vi "lab3_usrp_image_transceiver.vi"() -> ()   [LabVIEW 2014]
uses:
  glb_ackTable.vi
  var_stop.vi
  <vilib>/addons/Modulation/niDMT.lvlib
  <vilib>/addons/Modulation/Digital/General/MT Apply Pulse Shaping Filter (Generic).vi
  <vilib>/addons/Modulation/Analog/controls/Complex Data Waveform.ctl
  <vilib>/addons/Modulation/niAMT.lvlib
  <instrlib>/niUSRP/niUSRP Write Tx Data (CDB Cluster).vi
  <instrlib>/niUSRP/niUSRP Fetch Rx Data (CDB Cluster).vi
  <vilib>/addons/Modulation/Digital/General/MT Apply Matched Filter (Generic).vi
  <vilib>/addons/Modulation/Digital/General/MT Align to Ideal Symbols (Generic).vi
  glb_complete.vi
panel:
  in  "Debug":bool
  out "Constellation Graph":cdb[](graph)
  out "RX coerced gain":dbl format="%#_6f"
  out "TX coerced gain":dbl format="%#_6f"
  out "coerced carrier frequency":dbl=100000.0 format="%#_6p"
  out "coerced IQ rate":dbl=100000.0 format="%#_6p"
  out "Download progress":dbl(slide) scale=0.0..100.0
  out "Received Image":picture
  out "total bytes RX":i32
  in  "soft decision?":bool
  in  "RX number of samples":i64=40000
  in  "RX Frequency Source":string(combo)="Internal"
  in  "TX Frequency Source":string(combo)="Internal"
  in  "RX ant gain":dbl format="%#_6f"
  in  "TX ant gain":dbl format="%#_6f"
  in  "carrier frequency":dbl=915000000.0 format="%#_6p"
  in  "IQ rate":dbl=800000.0 format="%#_6p"
  in  "RX antenna name":string="RX2"
  in  "TX antenna name":string="TX1"
  in  "RX device names":refnum<k15>="192.168.10.2"
  in  "TX device names":refnum<k15>="192.168.10.2"
  in  "filter length (symbols)":i32=11
  in  "filter parameter":dbl=0.35 format="%.2f"
  in  "pulse shaping filter (none)":T1(ring)=enum."Root Raised Cos"
  in  "samples per symbol (16)":i32=4
  in  "Tab Control":T2(tab)=enum."r=1/2 (13,17)"
  in  "modulation 2":enum16{"BPSK", "QPSK"}(ring)
  in  "modulation 3":enum16{"BPSK", "QPSK"}(ring)=enum."QPSK"
  in  "modulation":enum16{"BPSK", "QPSK", "16QAM"}(ring)
  in  "stop":bool
  out "Length of last packet":i32
  out "total packets":dbl
  in  "bytes per packet":i32=1000
  out "Original image":picture
  out "Total bits TX":i32
  in  "file path (use dialog)":path
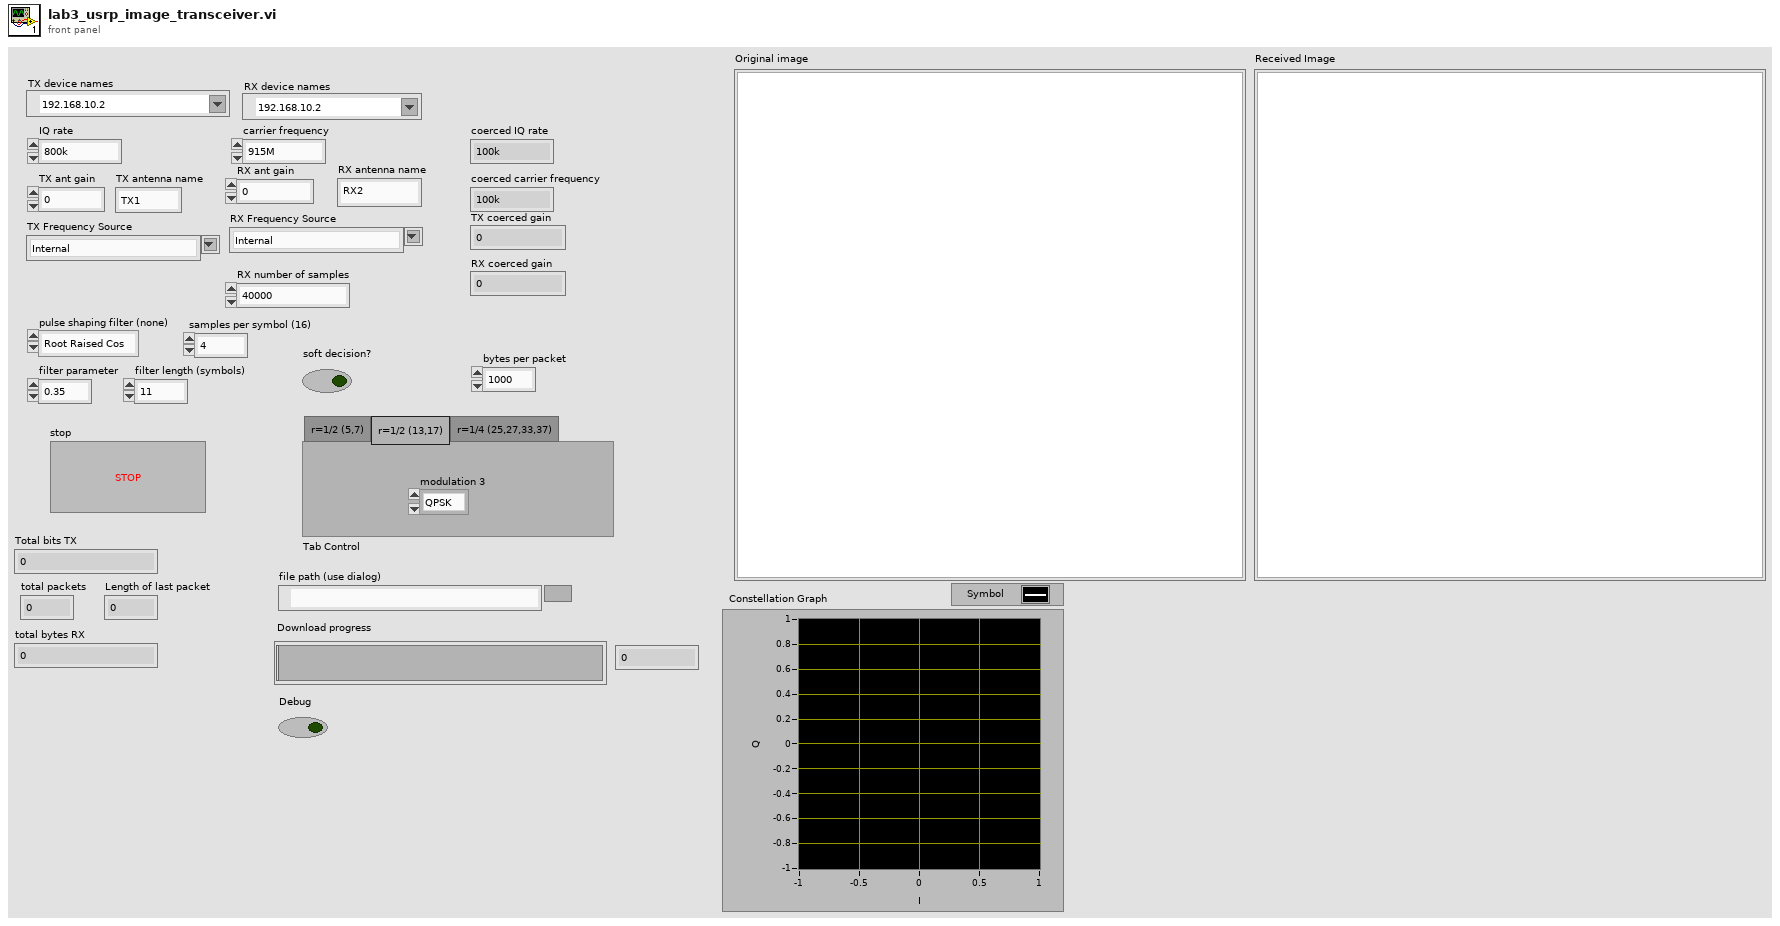
[diagram p1: front panel]
types:
  T1 = enum16{"none", "Raised Cosine", "Root Raised Cos", "Gaussian"}
  T2 = enum32{"r=1/2 (5,7)", "r=1/2 (13,17)", "r=1/4 (25,27,33,37)"}
  T3 = cluster{"use 24bit?":bool, "dimension":i32[], "top left":cluster{"x":i16, "y":i16}, "colors":u32[], "mask":u8[]}
  T4 = enum16{"FSK", "PSK", "QAM", "MSK", "PAM", "ASK", "CPM"}
  T5 = cluster{"counter":i32, "bitslength":i32, "bitstream":bool[]}
  T6 = enum16{"r=1/2 (5,7)", "r=1/2 (13,17)", "r=1/4 (25,27,33,37)"}
  T7 = typedef "niAMT.lvlib/Complex Data Waveform.ctl" = cluster{"t0":dbl, "dt":dbl, "Y":cdb[]}
  T8 = typedef "imagedata.ctl" = cluster{"image type":i32, "image depth":i32, "image":u8[], "mask":u8[], "colors":u32[], "Rectangle":cluster{"left":i16, "top":i16, "right":i16, "bottom":i16}}
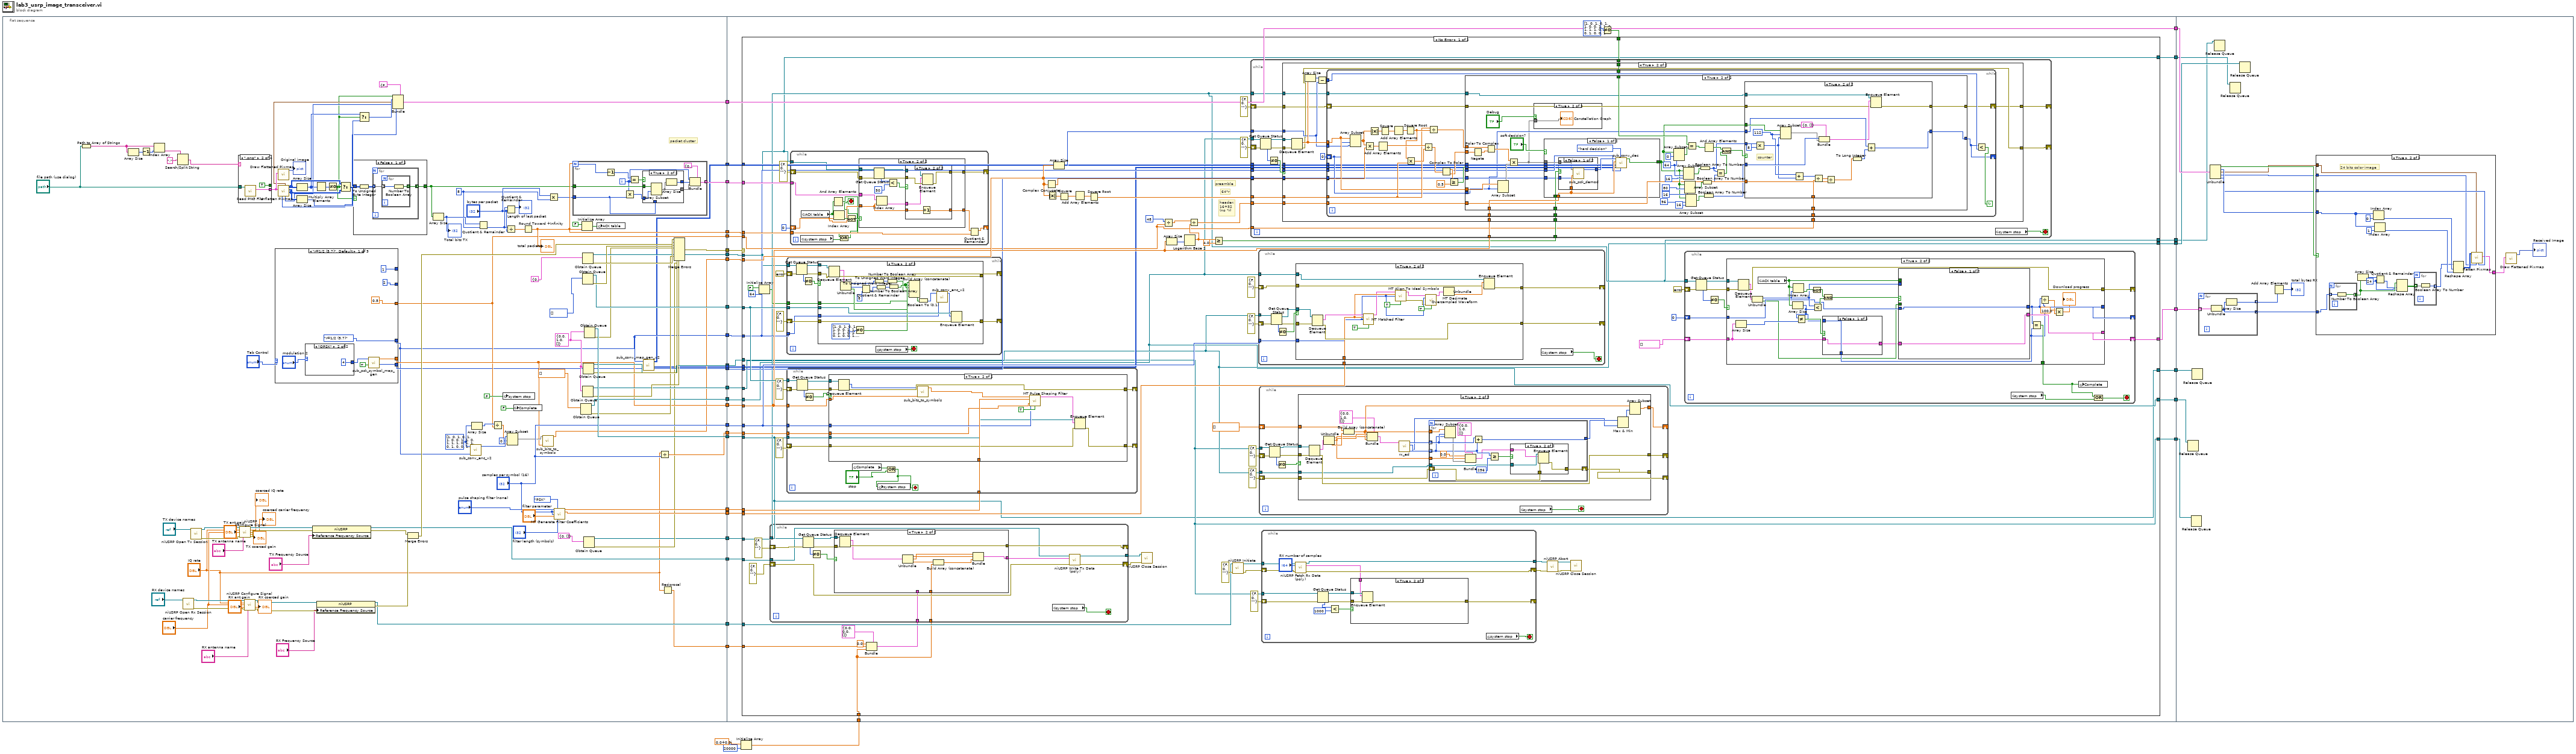
[diagram p0: block diagram]
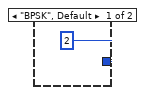
[diagram p2: hidden frame]
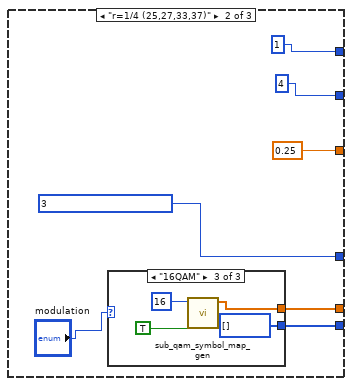
[diagram p3: hidden frame]
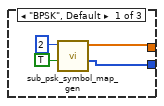
[diagram p4: hidden frame]
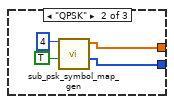
[diagram p5: hidden frame]
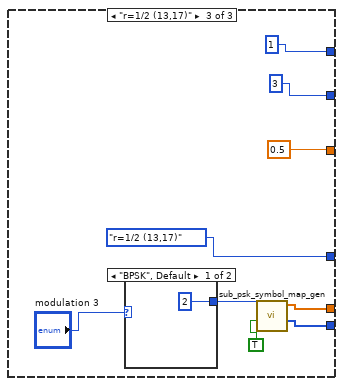
[diagram p6: hidden frame]
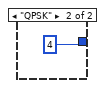
[diagram p7: hidden frame]
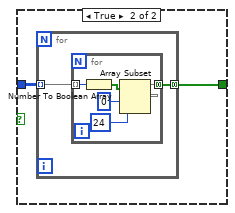
[diagram p8: hidden frame]
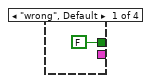
[diagram p9: hidden frame]
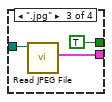
[diagram p10: hidden frame]
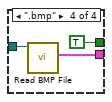
[diagram p11: hidden frame]
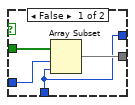
[diagram p12: hidden frame]
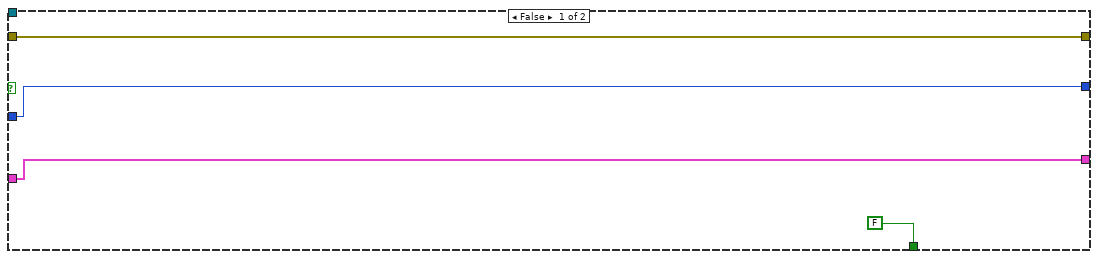
[diagram p13: hidden frame]
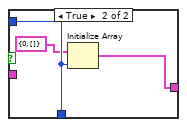
[diagram p14: hidden frame]
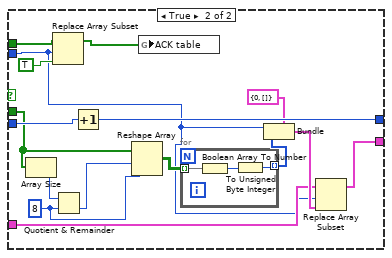
[diagram p15: hidden frame]
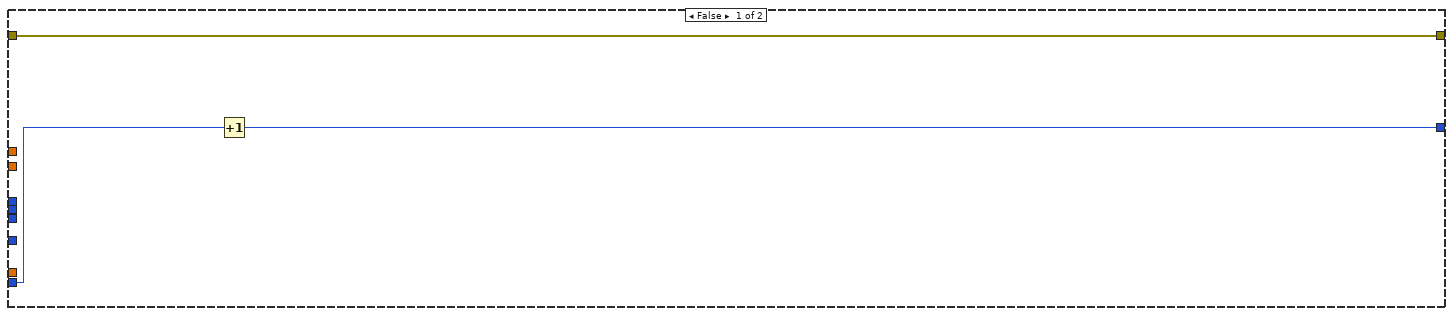
[diagram p17: hidden frame]
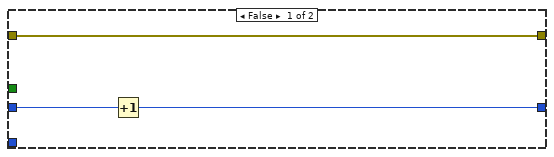
[diagram p19: hidden frame]
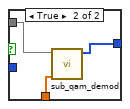
[diagram p20: hidden frame]
diagram:
  n1 = flat-sequence {
    tunnel: [w123] -> w36
    tunnel: [w119] -> w35
    tunnel: [w116] -> w34
    tunnel: [w115] -> w33
    tunnel: [w112] -> w32
    tunnel: [w41] -> w31
    tunnel: [w109] -> w30
    tunnel: [w104] -> w29
    tunnel: ["samples per symbol (16)"] -> w28
    tunnel: [w81] -> w27
    tunnel: [w80] -> w26
    tunnel: [w79] -> w25
    tunnel: [w77] -> w24
    tunnel: [w74] -> w23
    tunnel: [w73] -> w22
    tunnel: [w70] -> w21
    tunnel: [w63] -> w20
    tunnel: [w62] -> w19
    tunnel: [w61] -> w18
    tunnel: [w60] -> w17
    tunnel: [w57] -> w16
    tunnel: [w48] -> w13
    tunnel: [w42] -> w10
    tunnel: [w40] -> w8
    tunnel: [w39] -> w7
    tunnel: w36 -> [w262]
    tunnel: w35 -> [w263]
    tunnel: w34 -> [w260]
    tunnel: w33 -> [w259]
    tunnel: w32 -> [w257]
    tunnel: w31 -> [w256]
    tunnel: w30 -> [w247]
    tunnel: w29 -> [w248]
    tunnel: w28 -> [w250]
    tunnel: w27 -> [w249]
    tunnel: w26 -> [w244]
    tunnel: w25 -> [w243]
    tunnel: w24 -> [w255]
    tunnel: w23 -> [w253]
    tunnel: w22 -> [w246]
    tunnel: w21 -> [w252]
    tunnel: w20 -> [w251]
    tunnel: w19 -> [w258]
    tunnel: w18 -> [w261]
    tunnel: w17 -> [w254]
    tunnel: w16 -> [w245]
    tunnel: [w242] -> w15
    tunnel: [w239] -> w14
    tunnel: w13 -> [w239]
    tunnel: w11 -> [w238]
    tunnel: w10 -> [w237]
    tunnel: w8 -> [w236]
    tunnel: w7 -> [w235]
    tunnel: [w234] -> w6
    tunnel: [w233] -> w5
    tunnel: [w232] -> w4
    tunnel: [w231] -> w3
    tunnel: [w230] -> w2
    tunnel: [w229] -> w1
    tunnel: w15 -> [w841]
    tunnel: w14 -> [w840]
    tunnel: w6 -> [w829]
    tunnel: w5 -> [w831]
    tunnel: w4 -> [w830]
    tunnel: w3 -> [w828]
    tunnel: w2 -> [w827]
    tunnel: w1 -> [w826]
    frame #0 {
      w69 = i16[] [1, 0, 1, 0, 1, 1, 0, 0, 1, 1, 0, 1, 1, 1, 0, 1, 1, 0, 1, 0, 0, 1, 0, 0, 1, 1, 1, 0, 0, 0, 1, 0, 1, 1, 1, 1, 0, 0, 1, 0, 1, 0, 0, 0, 1, 1, 0, 0, 0, 0, 1, 0, 0, 0, 0, 0, 1, 1, 1, 1, 1, 1, 0, 0] ("preamble(64) 2")
      w76 = T7 {"t0"=0.0, "dt"=1.0, "Y"=[]} ("output complex waveform")
      w120 = 8 ("y")
      # "packet cluster"
      n2 = Path to Array of Strings(0:"file path (use dialog)") -> (2:w142:string[])  [unwired: 1 out]
      n3 = Array Size(array=w142) -> (size(s)=w141:i32)
      n4 = Decrement(x=w141) -> (x-1=w140:i32)
      n5 = Index Array(array=w142, index=w140) -> (element=w139:string)
      n6 = Search/Split String(string=w139, search string/char (-)=".") -> (match + rest of string=w137:string)  [unwired: 1 in, 2 out]
      n7 = call <instrlib>:"niUSRP Open Rx Session.vi"("device names"="RX device names") -> ("session handle out"=w97:refnum<k15>, "error out"=w96:errorcluster)  [unwired: 13 in]
      n8 = call <instrlib>:"niUSRP Open Tx Session.vi"("device names"="TX device names") -> ("session handle out"=w101:refnum<k15>, "error out"=w100:errorcluster)  [unwired: 13 in]
      n9 = case shown="\".png\"" w137 {
        tunnel: [FALSE TRUE TRUE TRUE] -> _
        tunnel: "file path (use dialog)" -> [_ w202 w205 w208]
        tunnel: [_ w201 w204 w207] -> w132
        frame "wrong", Default {
        }
        frame ".png" {
          n10 = call <vilib>:"Read PNG File.vi"("path to PNG file"=w202) -> ("image data"=w201:T8)  [unwired: 8 in, 2 out]
        }
        frame ".jpg" {
          n11 = call <vilib>:"Read JPEG File.vi"("path to JPEG file"=w205) -> ("image data"=w204:T8)  [unwired: 8 in, 2 out]
        }
        frame ".bmp" {
          n12 = call <vilib>:"Read BMP File.vi"("path to BMP file"=w208) -> ("image data"=w207:T8)  [unwired: 8 in, 2 out]
        }
      }
      n13 = call <instrlib>:"niUSRP Configure Signal.vi"("session handle"=w101, "IQ rate"="IQ rate", "carrier frequency"="carrier frequency", "gain"="TX ant gain", "error in (no error)"=w100, "active antenna"="TX antenna name") -> ("session handle out"=w89:refnum<k15>, "coerced IQ rate"=→"coerced IQ rate":dbl, "coerced carrier frequency"=→"coerced carrier frequency":dbl, "coerced gain"=→"TX coerced gain":dbl, "error out"=w90:errorcluster)  [unwired: 5 in]
      n14 = call <instrlib>:"niUSRP Configure Signal.vi"("session handle"=w97, "IQ rate"="IQ rate", "carrier frequency"="carrier frequency", "gain"="RX ant gain", "error in (no error)"=w96, "active antenna"="RX antenna name") -> ("session handle out"=w92:refnum<k15>, "coerced gain"=→"RX coerced gain":dbl, "error out"=w91:errorcluster)  [unwired: 5 in, 2 out]
      n15 = case shown="\"r=1/2 (5,7)\", Default" "Tab Control" {
        tunnel: [T6."r=1/2 (5,7)" ("code type") T6 3 ("code type") T6."r=1/2 (13,17)" ("code type")] -> w41
        tunnel: [w144 w158 w174] -> w63
        tunnel: [1 1 1] -> _
        tunnel: [2 4 3] -> _
        tunnel: [0.5 0.25 0.5] -> w61
        tunnel: [w143 w154 w173] -> w60
        frame "r=1/2 (5,7)", Default {
          n16 = case shown="\"QPSK\"" "modulation 2" {
            tunnel: [2 4] -> w145
            frame "BPSK", Default {
            }
            frame "QPSK" {
            }
          }
          n17 = call "sub_psk_symbol_map_gen.vi"("Gray code?"=TRUE, "M-PSK"=w145) -> ("index map"=w143:u32[], "symbol map"=w144:cdb[])  [unwired: 8 in]
        }
        frame "r=1/4 (25,27,33,37)" {
          n18 = case shown="\"16QAM\"" "modulation" {
            tunnel: [w162 w168 w172] -> w158
            tunnel: [w161 w167 u32[] [] ("index map")] -> w154
            frame "BPSK", Default {
              n19 = call "sub_psk_symbol_map_gen.vi"("Gray code?"=TRUE, "M-PSK"=2) -> ("index map"=w161:u32[], "symbol map"=w162:cdb[])  [unwired: 8 in]
            }
            frame "QPSK" {
              n20 = call "sub_psk_symbol_map_gen.vi"("Gray code?"=TRUE, "M-PSK"=4) -> ("index map"=w167:u32[], "symbol map"=w168:cdb[])  [unwired: 8 in]
            }
            frame "16QAM" {
              n21 = call "sub_qam_symbol_map_gen.vi"("Gray code?"=TRUE, "M-QAM"=16) -> ("symbol map"=w172:cdb[])  [unwired: 9 in]
            }
          }
        }
        frame "r=1/2 (13,17)" {
          n22 = case shown="\"BPSK\", Default" "modulation 3" {
            tunnel: [2 ("M-PSK") 4] -> w176
            frame "BPSK", Default {
            }
            frame "QPSK" {
            }
          }
          n23 = call "sub_psk_symbol_map_gen.vi"("Gray code?"=TRUE, "M-PSK"=w176) -> ("index map"=w173:u32[], "symbol map"=w174:cdb[])  [unwired: 8 in]
        }
      }
      n24 = call <vilib>:"Draw Flattened Pixmap.vi"("image data"=w132) -> ("new picture"=→"Original image":picture)  [unwired: 8 in]
      n25 = call <vilib>:"Unflatten Pixmap.vi"("image data"=w132) -> ("8-bit pixmap"=w134:u8[][], "24-bit pixmap"=w130:u32[][], "colors"=w51:u32[], "top left"=w52:cluster{"x":i16, "y":i16}, "mask"=w50:u8[])  [unwired: 4 in, 2 out]
      n26 = Array Size(array=w130) -> (size(s)=w55:i32[])
      n27 = Array Size(array=w134) -> (size(s)=w54:i32[])
      n28 = property class="niUSRP"(reference=w89, error in=w90, "Reference Frequency Source"="TX Frequency Source") -> (reference out=w80:refnum<k15>, error out=w86:errorcluster)
      n29 = Multiply Array Elements(1:w55) -> (0:w135:i32)
      n30 = property class="niUSRP"(reference=w92, error in=w91, "Reference Frequency Source"="RX Frequency Source") -> (reference out=w79:refnum<k15>, error out=w85:errorcluster)
      n31 = Not Equal To 0?(x=w135) -> (x != 0?=w38:bool)
      n32 = Select(t=w130, s=w38, f=w134) -> (s? t:f=w133:u32[][])
      n33 = case shown="False" w38 {
        tunnel: w133 -> [w186 w192]
        tunnel: [w184 w191] -> w122
        frame False {
          n34 = To Unsigned Byte Integer(number=w186) -> (unsigned 8bit integer=w185:u8[][])
          n35 = for {
            tunnel: w185 -> [w188] mode=indexing
            tunnel: [w187] -> w184 mode=concatenating
            n36 = for {
              tunnel: w188 -> [w190] mode=indexing
              tunnel: [w189] -> w187 mode=concatenating
              n37 = Number To Boolean Array(number=w190) -> (Boolean array=w189:bool[])
            }
          }
        }
        frame True {
          n38 = for {
            tunnel: w192 -> [w194] mode=indexing
            tunnel: [w193] -> w191 mode=concatenating
            n39 = for {
              tunnel: w194 -> [w199] mode=indexing
              tunnel: [w197] -> w193 mode=concatenating
              n40 = Number To Boolean Array(number=w199) -> (Boolean array=w198:bool[])
              n41 = Array Subset(array=w198, index=0, length=24) -> (w197:bool[])
            }
          }
        }
      }
      n42 = Select(t=w55, s=w38, f=w54) -> (s? t:f=w53:i32[])
      n43 = Bundle(cluster=T3 {"use 24bit?"=FALSE, "dimension"=[], "top left"={"x"=0, "y"=0}, "colors"=[], "mask"=[]}, "use 24bit?"=w38, "dimension"=w53, "top left"=w52, "colors"=w51, "mask"=w50) -> (w48:T3)
      n44 = Merge Errors(w86, w85) -> (w84:errorcluster)
      n45 = Array Size(array=w122) -> (size(s)=w128:i32)
      "Total bits TX" <- w128
      n46 = call "sub_conv_enc_v2.vi"("code type"=w41, "bitstream"=w69) -> ("coded bits"=w67:i16[])  [unwired: 9 in]
      n47 = Array Size(array=w69) -> (size(s)=w68:i32)
      n48 = Quotient & Remainder(x=w128, y=w120) -> (floor(x/y)=w127:i32)  [unwired: 1 out]
      n49 = Divide(x=w68, y=w61) -> (x/y=w66:dbl)
      n50 = global write "var_stop.vi" "system stop"(FALSE) -> ()
      n51 = Divide(x=w127, y="bytes per packet") -> (x/y=w129:dbl)
      n52 = Quotient & Remainder(x=w127, y="bytes per packet") -> (x-y*floor(x/y)=→"Length of last packet":i32)  [unwired: 1 out]
      n53 = Array Subset(array=w67, index=0, length=w66) -> (w64:i16[])
      n54 = global write "glb_complete.vi" "Complete"(FALSE) -> ()
      n55 = Round Toward +Infinity(x=w129) -> (ceil(x): smallest int >= x=w123:dbl)
      "total packets" <- w123
      n56 = call "sub_bits_to_symbols.vi"("symbol map"=w63, "bits"=w64) -> ("symbols"=w62:cdb[])  [unwired: 9 in]
      n57 = Multiply(x="bytes per packet", y=w120) -> (x*y=w37:i32)
      n58 = call <vilib>:"MT Generate Filter Coefficients.vi"("pulse shaping filter (none)"="pulse shaping filter (none)", "modulation type"=T4."PSK", "pulse shaping samples per symbol (16)"="samples per symbol (16)", "matched samples per symbol (16)"="samples per symbol (16)", "filter parameter"="filter parameter", "filter length (symbols)"="filter length (symbols)") -> ("pulse shaping filter coefficients"=w109:dbl[], "matched filter coefficients"=w73:dbl[])  [unwired: 7 in, 1 out]
      n59 = for {
        N: w123 -> [w220]
        tunnel: w122 -> [w217]
        tunnel: [w214] -> w119 mode=indexing
        tunnel: w37 -> [w210]
        i -> [w212]
        n60 = Decrement(x=w220) -> (x-1=w219:i32)
        n61 = Multiply(x=w212, y=w210) -> (x*y=w211:i32)
        n62 = Equal?(x=w219, y=w212) -> (x = y?=w218:bool)
        n63 = case shown="True" w218 {
          tunnel: w217 -> [w224 w228]
          tunnel: [w223 w226] -> w216
          tunnel: [w221 w227] -> w215
          tunnel: w211 -> [w222 w225]
          tunnel: w210 -> [w221 _]
          frame False {
            n64 = Array Subset(array=w224, index=w222, length=w221) -> (w223:bool[])
          }
          frame True {
            n65 = Array Subset(array=w228, index=w225) -> (w226:bool[])  [unwired: 1 in]
            n66 = Array Size(array=w226) -> (size(s)=w227:i32)
          }
        }
        n67 = Bundle(cluster=T5 {"counter"=0, "bitslength"=0, "bitstream"=[]}, "counter"=w212, "bitslength"=w215, "bitstream"=w216) -> (w214:T5)
      }
      n68 = Obtain Queue(element data type=cdb[] []) -> (queue out=w70:refnum<queue>, error out=w71:errorcluster)  [unwired: 4 in, 1 out]
      n69 = Initialize Array(FALSE, w123) -> (w124:bool[])
      n70 = Obtain Queue(element data type=T5 {"counter"=0, "bitslength"=0, "bitstream"=[]} ("cluster")) -> (queue out=w115:refnum<queue>, error out=w118:errorcluster)  [unwired: 4 in, 1 out]
      n71 = Obtain Queue(element data type=i32[] []) -> (queue out=w112:refnum<queue>, error out=w117:errorcluster)  [unwired: 4 in, 1 out]
      n72 = Obtain Queue(element data type=w76) -> (queue out=w74:refnum<queue>, error out=w75:errorcluster)  [unwired: 4 in, 1 out]
      n73 = Obtain Queue(element data type=w76) -> (queue out=w77:refnum<queue>, error out=w78:errorcluster)  [unwired: 4 in, 1 out]
      n74 = Obtain Queue(element data type=cluster{"counter":u32, "bitstream":bool[]} {"counter"=0, "bitstream"=[]} ("cluster")) -> (queue out=w57:refnum<queue>, error out=w58:errorcluster)  [unwired: 4 in, 1 out]
      n75 = Obtain Queue(element data type=w76) -> (queue out=w104:refnum<queue>, error out=w83:errorcluster)  [unwired: 4 in, 1 out]
      n76 = global write "glb_ackTable.vi" "ACK table"(w124) -> ()
      n77 = call "sub_conv_map_gen_v2.vi"("code type"=w41) -> ("output in decimal"=w39:u32[][], "state transition"=w40:u32[][])  [unwired: 9 in]
      n78 = Divide(x="IQ rate", y="samples per symbol (16)") -> (x/y=w81:dbl)
      n79 = Reciprocal(x="IQ rate") -> (1/x=w42:dbl)
      n80 = Merge Errors(w118, w117, w84, w83, w78, w75, w71, w58) -> (w116:errorcluster)
    }
    frame #1 {
      n81 = Not Equal To 0?(x=i16[] [1, 0, 1, 0, 1, 1, 0, 0, 1, 1, 0, 1, 1, 1, 0, 1, 1, 0, 1, 0, 0, 1, 0, 0, 1, 1, 1, 0, 0, 0, 1, 0, 1, 1, 1, 1, 0, 0, 1, 0, 1, 0, 0, 0, 1, 1, 0, 0, 0, 0, 1, 0, 0, 0, 0, 0, 1, 1, 1, 1, 1, 1, 0, 0] ("preamble(64) 2")) -> (x != 0?=w240:bool[])
      n82 = case shown="No Error" w260 {
        tunnel: w262 -> [w335 _]
        tunnel: w263 -> [w334 _]
        tunnel: w259 -> [w268 w825]
        tunnel: w257 -> [w330 _]
        tunnel: w256 -> [w288 _]
        tunnel: w251 -> [w296 _]
        tunnel: w247 -> [w328 _]
        tunnel: w250 -> [w307 _]
        tunnel: w248 -> [w265 w823]
        tunnel: w249 -> [w326 _]
        tunnel: w244 -> [w325 _]
        tunnel: w243 -> [w314 _]
        tunnel: w255 -> [w266 w820]
        tunnel: w253 -> [w269 w824]
        tunnel: w246 -> [w308 _]
        tunnel: w252 -> [w267 w821]
        tunnel: w258 -> [w301 _]
        tunnel: w261 -> [w286 _]
        tunnel: w254 -> [w292 _]
        tunnel: w240 -> [w287 _]
        tunnel: w245 -> [w270 w822]
        tunnel: [w282 _] -> w242
        tunnel: w238 -> [w264 _]
        tunnel: w237 -> [w279 _]
        tunnel: w236 -> [w276 _]
        tunnel: w235 -> [w275 _]
        tunnel: [w270 w822] -> w234
        tunnel: [w269 w824] -> w233
        tunnel: [w268 w825] -> w232
        tunnel: [w266 w823] -> w231
        tunnel: [w267 w821] -> w230
        tunnel: [w265 w820] -> w229
        frame No Error {
          # "header:\n16+32\n(no *r)"
          # "64*r"
          # "preamble"
          n83 = Initialize Array(FALSE, 64 ("dimension size")) -> (w271:bool[])
          n84 = while {
            tunnel: w330 -> [w729]
            shift-right: [w723] -> _
            shift-left: errorcluster {"status"=FALSE, "code"=0, "source"=""} ("error out") -> [w724]
            tunnel: w296 -> [w722]
            tunnel: w328 -> [w721]
            tunnel: w307 -> [w720]
            tunnel: w265 -> [w719]
            shift-right: [w717] -> _
            shift-left: errorcluster {"status"=FALSE, "code"=0, "source"=""} ("error out") -> [w718]
            tunnel: w326 -> [w716]
            stop <- w713 stop-if-true
            n85 = Get Queue Status(queue=w729, error in (no error)=w724) -> (queue out=w726:refnum<queue>, error out=w725:errorcluster, # elements in queue=w728:i32)  [unwired: 1 in, 5 out]
            n86 = Not Equal To 0?(x=w728) -> (x != 0?=w727:bool)
            n87 = case shown="True" w727 {
              tunnel: w726 -> [_ w745]
              tunnel: w725 -> [w731 w744]
              tunnel: [w731 w743] -> w723
              tunnel: w722 -> [_ w741]
              tunnel: w721 -> [_ w739]
              tunnel: w720 -> [_ w738]
              tunnel: w719 -> [_ w736]
              tunnel: w718 -> [w730 w735]
              tunnel: [w730 w734] -> w717
              tunnel: w716 -> [_ w733]
              frame False {
              }
              frame True {
                n88 = Dequeue Element(queue=w745, error in (no error)=w744) -> (element=w742:i32[], error out=w743:errorcluster)  [unwired: 1 in, 2 out]
                n89 = call "sub_bits_to_symbols.vi"("symbol map"=w741, "bits"=w742) -> ("symbols"=w732:cdb[])  [unwired: 9 in]
                n90 = call-poly <vilib>:"MT Pulse Shaping Filter.vi"("symbols"=w732, "pulse shaping filter coefficients"=w739, "samples per symbol (16)"=w738, "symbol rate (Hz)"=w733, "reset? (T)"=TRUE) -> ("output complex waveform"=w737:T7)  [unwired: 9 in, 1 out]
                n91 = Enqueue Element(queue=w736, element=w737, error in (no error)=w735) -> (error out=w734:errorcluster)  [unwired: 1 in, 2 out]
              }
            }
            n92 = global read "glb_complete.vi" "Complete"() -> (w715:bool)
            n93 = Compound Arithmetic op=OR(w715, "stop") -> (w713:bool)
            n94 = global write "var_stop.vi" "system stop"(w713) -> ()
          }
          n95 = while {
            tunnel: w268 -> [w758]
            shift-right: [w752] -> _
            shift-left: errorcluster {"status"=FALSE, "code"=0, "source"=""} ("error out") -> [w756]
            tunnel: w330 -> [w750]
            shift-right: [w749] -> _
            shift-left: errorcluster {"status"=FALSE, "code"=0, "source"=""} ("error out") -> [w748]
            tunnel: w288 -> [w747]
            tunnel: w271 -> [w746]
            stop <- w751 stop-if-true
            n96 = Get Queue Status(queue=w758, error in (no error)=w756) -> (queue out=w754:refnum<queue>, error out=w753:errorcluster, # elements in queue=w757:i32)  [unwired: 1 in, 5 out]
            n97 = Not Equal To 0?(x=w757) -> (x != 0?=w755:bool)
            n98 = case shown="True" w755 {
              tunnel: w754 -> [_ w783]
              tunnel: w753 -> [w760 w782]
              tunnel: [w760 w781] -> w752
              tunnel: w750 -> [_ w779]
              tunnel: [w759 w778] -> w749
              tunnel: w748 -> [w759 w777]
              tunnel: w747 -> [_ w763]
              tunnel: w746 -> [_ w761]
              frame False {
              }
              frame True {
                n99 = Dequeue Element(queue=w783, error in (no error)=w782) -> (element=w780:T5, error out=w781:errorcluster)  [unwired: 1 in, 2 out]
                n100 = Unbundle(w780) -> ("counter"=w774:i32, "bitslength"=w776:i32, "bitstream"=w767:bool[])
                n101 = Not Equal To 0?(x=i16[] [1, 0, 1, 0, 1, 1, 0, 0, 1, 1, 0, 1, 1, 1, 0, 1, 1, 0, 1, 0, 0, 1, 0, 0, 1, 1, 1, 0, 0, 0, 1, 0, 1, 1, 1, 1, 0, 0, 1, 0, 1, 0, 0, 0, 1, 1, 0, 0, 0, 0, 1, 0, 0, 0, 0, 0, 1, 1, 1, 1, 1, 1, 0, 0] ("preamble(64) 2")) -> (x != 0?=w770:bool[])
                n102 = Quotient & Remainder(x=w776, y=8) -> (floor(x/y)=w762:i32)  [unwired: 1 out]
                n103 = To Unsigned Word Integer(number=w774) -> (unsigned 16bit integer=w772:u16)
                n104 = To Unsigned Word Integer(number=w762) -> (unsigned 16bit integer=w771:u16)
                n105 = Number To Boolean Array(number=w772) -> (Boolean array=w768:bool[])
                n106 = Number To Boolean Array(number=w771) -> (Boolean array=w769:bool[])
                n107 = Build Array (concatenate)(w770, w769, w769, w768, w767, w761) -> (w766:bool[])
                n108 = Boolean To (0,1)(Boolean=w766) -> (0, 1=w765:i16[])
                n109 = call "sub_conv_enc_v2.vi"("code type"=w763, "bitstream"=w765) -> ("coded bits"=w764:i16[])  [unwired: 9 in]
                n110 = Enqueue Element(queue=w779, element=w764, error in (no error)=w777) -> (error out=w778:errorcluster)  [unwired: 1 in, 2 out]
              }
            }
            n111 = global read "var_stop.vi" "system stop"() -> (w751:bool)
          }
          n112 = while {
            tunnel: w335 -> [w797]
            shift-right: [w796] -> _
            shift-left: 0 -> [w790]
            tunnel: w334 -> [w791]
            tunnel: w268 -> [w792]
            shift-right: [w788] -> _
            shift-left: errorcluster {"status"=FALSE, "code"=0, "source"=""} ("error out") -> [w789]
            stop <- w784 stop-if-true
            n113 = global read "var_stop.vi" "system stop"() -> (w786:bool)
            n114 = global read "glb_ackTable.vi" "ACK table"() -> (w793:bool[])
            n115 = And Array Elements(Boolean array=w793) -> (logical AND=w785:bool)
            n116 = Index Array(array=w793, index=w790) -> (element=w795:bool)
            n117 = Compound Arithmetic op=OR(w785, w786) -> (w784:bool)
            n118 = Not(x=w795) -> (.not. x?=w794:bool)
            n119 = case shown="True" w794 {
              tunnel: w792 -> [_ w811]
              tunnel: w791 -> [_ w805]
              tunnel: w790 -> [w798 w801]
              tunnel: w789 -> [w799 w803]
              tunnel: [w799 w802] -> w788
              tunnel: [w798 w800] -> w787
              frame False {
              }
              frame True {
                n120 = Get Queue Status(queue=w811, error in (no error)=w803) -> (queue out=w808:refnum<queue>, error out=w807:errorcluster, # elements in queue=w810:i32)  [unwired: 1 in, 5 out]
                n121 = Index Array(array=w805, index=w801) -> (element=w804:T5)
                n122 = Less?(x=w810, y=50 ("# elements in queue")) -> (x < y?=w809:bool)
                n123 = case shown="True" w809 {
                  tunnel: w808 -> [_ w819]
                  tunnel: w807 -> [w813 w818]
                  tunnel: w804 -> [_ w817]
                  tunnel: [w813 w816] -> w802
                  tunnel: w801 -> [w812 w815]
                  tunnel: [w812 w814] -> w800
                  frame False {
                  }
                  frame True {
                    n124 = Increment(x=w815) -> (x+1=w814:dbl)
                    n125 = Enqueue Element(queue=w819, element=w817, error in (no error)=w818) -> (error out=w816:errorcluster)  [unwired: 1 in, 2 out]
                  }
                }
              }
            }
            n126 = Quotient & Remainder(x=w787, y=w797) -> (x-y*floor(x/y)=w796:dbl)  [unwired: 1 out]
          }
          n127 = Bundle(cluster=T7 {"t0"=0.0, "dt"=0.0, "Y"=[]} ("output complex waveform"), "t0"=0.0, "dt"=w279, "Y"=w264) -> (w277:T7)
          n128 = while {
            tunnel: w265 -> [w700]
            shift-right: [w695] -> _
            shift-left: errorcluster {"status"=FALSE, "code"=0, "source"=""} ("error out") -> [w699]
            tunnel: w325 -> [w693]
            shift-right: [w692] -> w323
            shift-left: errorcluster {"status"=FALSE, "code"=0, "source"=""} ("error out") -> [w691]
            tunnel: [w690] -> w322
            tunnel: w277 -> [w687]
            tunnel: w264 -> [w686]
            stop <- w694 stop-if-true
            n129 = Get Queue Status(queue=w700, error in (no error)=w699) -> (queue out=w697:refnum<queue>, error out=w696:errorcluster, # elements in queue=w698:i32)  [unwired: 1 in, 5 out]
            n130 = Not Equal To 0?(x=w698) -> (x != 0?=w688:bool)
            n131 = case shown="True" w688 {
              tunnel: w697 -> [_ w712]
              tunnel: w696 -> [w702 w711]
              tunnel: [w702 w710] -> w695
              tunnel: [w701 w703] -> w689
              tunnel: w687 -> [w701 _]
              tunnel: w686 -> [_ w707]
              frame False {
              }
              frame True {
                n132 = Dequeue Element(queue=w712, error in (no error)=w711) -> (element=w709:T7, error out=w710:errorcluster)  [unwired: 1 in, 2 out]
                n133 = Unbundle(w709) -> ("t0"=w704:dbl, "dt"=w705:dbl, "Y"=w708:cdb[])
                n134 = Build Array (concatenate)(w708, w707) -> (w706:cdb[])
                n135 = Bundle("t0"=w704, "dt"=w705, w706) -> (w703:cluster{"t0":dbl, "dt":dbl, cdb[]})  [unwired: 1 in]
              }
            }
            n136 = global read "var_stop.vi" "system stop"() -> (w694:bool)
            n137 = call-poly <instrlib>:"niUSRP Write Tx Data (poly).vi"("session handle"=w693, "data"=w689, "error in (no error)"=w691) -> ("session handle out"=w690:refnum<k15>, "error out"=w692:errorcluster)  [unwired: 11 in]
          }
          n138 = Complex Conjugate(1:w301) -> (0:w299:cdb[])
          n139 = Absolute Value(x=w301) -> (abs(x)=w304:dbl[])
          n140 = Array Size(array=w301) -> (size(s)=w300:i32)
          n141 = Square(x=w304) -> (x^2=w303:dbl[])
          n142 = Add Array Elements(numeric array=w303) -> (sum=w302:dbl)
          n143 = Square Root(x=w302) -> (sqrt(x)=w298:dbl)
          n144 = call <instrlib>:"niUSRP Close Session.vi"("session handle"=w322, "error in (no error)"=w323) -> ()  [unwired: 13 in, 1 out]
          n145 = Divide(x=48, y=w286) -> (x/y=w291:dbl)
          n146 = Array Size(array=w296) -> (size(s)=w295:i32)
          n147 = Logarithm Base 2(1:w295) -> (0:w290:dbl)
          n148 = Divide(x=w291, y=w290) -> (x/y=w289:dbl)
          n149 = Greater Or Equal?(x=w290, y=4.0) -> (x >= y?=w293:bool)
          n150 = call <instrlib>:"niUSRP Initiate.vi"("session handle"=w314, "error in (no error)"=errorcluster {"status"=FALSE, "code"=0, "source"=""}) -> ("session handle out"=w318:refnum<k15>, "error out"=w319:errorcluster)  [unwired: 12 in]
          n151 = while {
            tunnel: w267 -> [w427]
            shift-right: [w421] -> _
            shift-left: errorcluster {"status"=FALSE, "code"=0, "source"=""} ("error out") -> [w426]
            tunnel: w300 -> [w420]
            tunnel: w299 -> [w419]
            tunnel: w298 -> [w418]
            tunnel: w296 -> [w416]
            tunnel: w293 -> [w415]
            tunnel: w292 -> [w414]
            tunnel: w289 -> [w413]
            tunnel: w288 -> [w412]
            tunnel: w287 -> [w411]
            tunnel: w286 -> [w410]
            tunnel: w270 -> [w409]
            shift-right: [w408] -> _
            shift-left: errorcluster {"status"=FALSE, "code"=0, "source"=""} ("error out") -> [w407]
            tunnel: w276 -> [w406]
            tunnel: w275 -> [w405]
            stop <- w417 stop-if-true
            n152 = Get Queue Status(queue=w427, error in (no error)=w426) -> (queue out=w422:refnum<queue>, error out=w423:errorcluster, # elements in queue=w425:i32)  [unwired: 1 in, 5 out]
            n153 = Not Equal To 0?(x=w425) -> (x != 0?=w424:bool)
            n154 = case shown="True" w424 {
              tunnel: w423 -> [w429 w451]
              tunnel: w422 -> [_ w450]
              tunnel: [w429 w435] -> w421
              tunnel: w420 -> [_ w445]
              tunnel: w419 -> [_ w444]
              tunnel: w418 -> [_ w443]
              tunnel: w416 -> [_ w442]
              tunnel: w415 -> [_ w441]
              tunnel: w414 -> [_ w440]
              tunnel: w413 -> [_ w439]
              tunnel: w412 -> [_ w438]
              tunnel: w411 -> [_ w437]
              tunnel: w410 -> [_ w436]
              tunnel: w409 -> [_ w434]
              tunnel: [w428 w433] -> w408
              tunnel: w407 -> [w428 w432]
              tunnel: w406 -> [_ w431]
              tunnel: w405 -> [_ w430]
              frame False {
              }
              frame True {
                n155 = Dequeue Element(queue=w450, error in (no error)=w451) -> (element=w448:cdb[], error out=w435:errorcluster)  [unwired: 1 in, 2 out]
                n156 = Array Size(array=w448) -> (size(s)=w447:i32)
                n157 = Subtract(x=w447, y=w445) -> (x-y=w446:i32)
                n158 = while {
                  tunnel: w448 -> [w466]
                  shift-right: [w469] -> _
                  shift-left: 0 -> [w465]
                  tunnel: w446 -> [w471]
                  tunnel: w445 -> [w464]
                  tunnel: w444 -> [w485]
                  tunnel: w443 -> [w473]
                  tunnel: w442 -> [w463]
                  tunnel: w441 -> [w462]
                  tunnel: w440 -> [w461]
                  tunnel: w439 -> [w460]
                  tunnel: w438 -> [w459]
                  tunnel: w437 -> [w458]
                  tunnel: w436 -> [w457]
                  tunnel: w434 -> [w456]
                  shift-right: [w455] -> w433
                  shift-left: w432 -> [w454]
                  tunnel: w431 -> [w453]
                  tunnel: w430 -> [w452]
                  stop <- w470 continue-if-true
                  n159 = Array Subset(array=w466, index=w465, length=w464) -> (w481:cdb[])
                  n160 = Multiply(x=w481, y=w485) -> (x*y=w484:cdb[])
                  n161 = Absolute Value(x=w481) -> (abs(x)=w480:dbl[])
                  n162 = Add Array Elements(numeric array=w484) -> (sum=w477:cdb)
                  n163 = Square(x=w480) -> (x^2=w479:dbl[])
                  n164 = Add Array Elements(numeric array=w479) -> (sum=w478:dbl)
                  n165 = Square Root(x=w478) -> (sqrt(x)=w474:dbl)
                  n166 = Multiply(x=w474, y=w473) -> (x*y=w476:dbl)
                  n167 = Divide(x=w477, y=w476) -> (x/y=w475:cdb)
                  n168 = Divide(x=w473, y=w474) -> (x/y=w467:dbl)
                  n169 = Complex To Polar(r * e^(i*theta)=w475) -> (r=w483:dbl, theta=w468:dbl)
                  n170 = Greater Or Equal?(x=w483, y=0.5) -> (x >= y?=w472:bool)
                  n171 = case shown="True" w472 {
                    tunnel: [w488 w502] -> w469
                    tunnel: w468 -> [_ w530]
                    tunnel: w467 -> [_ w528]
                    tunnel: w466 -> [_ w527]
                    tunnel: w465 -> [w486 w491]
                    tunnel: w463 -> [_ w524]
                    tunnel: w462 -> [_ w523]
                    tunnel: w461 -> [_ w522]
                    tunnel: w460 -> [_ w500]
                    tunnel: w459 -> [_ w520]
                    tunnel: w458 -> [_ w517]
                    tunnel: w457 -> [_ w501]
                    tunnel: w456 -> [_ w499]
                    tunnel: [w487 w498] -> w455
                    tunnel: w454 -> [w487 w497]
                    tunnel: w453 -> [_ w493]
                    tunnel: w452 -> [_ w492]
                    frame False {
                      n172 = Increment(x=w486) -> (x+1=w488:i32)
                    }
                    frame True {
                      w516 = 64 ("length")
                      n173 = Negate(x=w530) -> (-x=w529:dbl)
                      n174 = Polar To Complex(1:w529, 2:w528) -> (0:w526:cdb)
                      n175 = Array Subset(array=w527, index=w491) -> (w525:cdb[])  [unwired: 1 in]
                      n176 = Multiply(x=w526, y=w525) -> (x*y=w489:cdb[])
                      n177 = case shown="True" "Debug" {
                        tunnel: w489 -> [_ w531]
                        frame False {
                        }
                        frame True {
                          "Constellation Graph" <- w531
                        }
                      }
                      n178 = case shown="False" "soft decision?" {
                        tunnel: w524 -> [w559 w577]
                        tunnel: w523 -> [w564 _]
                        tunnel: w489 -> [w563 w578]
                        tunnel: w522 -> [w562 _]
                        tunnel: w520 -> [w557 w574]
                        tunnel: [w558 w575] -> w503
                        tunnel: w493 -> [w556 w573]
                        tunnel: w492 -> [w555 w572]
                        frame False {
                          n179 = case shown="False" w564 {
                            tunnel: w563 -> [w568 w571]
                            tunnel: w559 -> [w567 w570]
                            tunnel: w562 -> [w566 _]
                            tunnel: [w565 w569] -> w561
                            frame False {
                              n180 = call "sub_psk_demod.vi"("index map"=w566, "symbol map"=w567, "symbol"=w568) -> ("bitstream"=w565:i16[])  [unwired: 8 in]
                            }
                            frame True {
                              n181 = call "sub_qam_demod.vi"("symbol map"=w570, "symbol"=w571) -> ("bitstream"=w569:i16[])  [unwired: 9 in]
                            }
                          }
                          n182 = call "sub_conv_dec.vi"("code type"=w557, "decision type"=enum16{"hard decision", "soft decision"}."hard decision", "output in decimal"=w555, "state transition"=w556, "symbol map"=w559, "hard bits/soft symbols"=w561) -> ("Decoded"=w558:bool[])  [unwired: 5 in]
                        }
                        frame True {
                          n183 = call "sub_conv_dec.vi"("code type"=w574, "decision type"=enum16{"hard decision", "soft decision"}."soft decision", "output in decimal"=w572, "state transition"=w573, "symbol map"=w577, "hard bits/soft symbols"=w578) -> ("Decoded"=w575:bool[])  [unwired: 5 in]
                        }
                      }
                      n184 = Array Subset(array=w503, index=0, length=w516) -> (w518:bool[])
                      n185 = Array Subset(array=w503, index=w516, length=16) -> (w508:bool[])
                      n186 = Array Subset(array=w503, index=80, length=16) -> (w509:bool[])
                      n187 = Array Subset(array=w503, index=96, length=16) -> (w510:bool[])
                      n188 = Equal?(x=w517, y=w518) -> (x = y?=w506:bool[])
                      n189 = Boolean Array To Number(Boolean array=w508) -> (number=w496:u32)
                      n190 = Boolean Array To Number(Boolean array=w509) -> (number=w495:u32)
                      n191 = And Array Elements(Boolean array=w506) -> (logical AND=w505:bool)
                      n192 = Boolean Array To Number(Boolean array=w510) -> (number=w494:u32)
                      n193 = Equal?(x=w496, y=w495) -> (x = y?=w507:bool)
                      n194 = And(x=w505, y=w507) -> (x .and. y?=w504:bool)
                      n195 = case shown="True" w504 {
                        tunnel: w503 -> [_ w554]
                        tunnel: w494 -> [_ w551]
                        tunnel: w496 -> [_ w553]
                        tunnel: w491 -> [w534 w543]
                        tunnel: [w533 w542] -> w502
                        tunnel: w501 -> [_ w546]
                        tunnel: w500 -> [_ w544]
                        tunnel: w499 -> [_ w539]
                        tunnel: [w532 w537] -> w498
                        tunnel: w497 -> [w532 w536]
                        frame False {
                          n196 = Increment(x=w534) -> (x+1=w533:i32)
                        }
                        frame True {
                          w549 = 112 ("index")
                          # "counter"
                          n197 = Multiply(x=w553, y=u32 8) -> (x*y=w548:u32)
                          n198 = Array Subset(array=w554, index=w549, length=w548) -> (w535:bool[])
                          n199 = Add(x=w549, y=w548) -> (x+y=w547:u32)
                          n200 = Divide(x=w547, y=w546) -> (x/y=w545:dbl)
                          n201 = Bundle(cluster=cluster{"counter":u32, "bitstream":bool[]} {"counter"=0, "bitstream"=[]}, "counter"=w551, "bitstream"=w535) -> (w538:cluster{"counter":u32, "bitstream":bool[]})
                          n202 = Divide(x=w545, y=w544) -> (x/y=w541:dbl)
                          n203 = To Long Integer(number=w541) -> (32bit integer=w540:i32)
                          n204 = Add(x=w543, y=w540) -> (x+y=w542:i32)
                          n205 = Enqueue Element(queue=w539, element=w538, error in (no error)=w536) -> (error out=w537:errorcluster)  [unwired: 1 in, 2 out]
                        }
                      }
                    }
                  }
                  n206 = Less?(x=w469, y=w471) -> (x < y?=w470:bool)
                }
              }
            }
            n207 = global read "var_stop.vi" "system stop"() -> (w417:bool)
          }
          n208 = while {
            tunnel: w269 -> [w591]
            shift-right: [w585] -> _
            shift-left: errorcluster {"status"=FALSE, "code"=0, "source"=""} ("error out") -> [w590]
            tunnel: w308 -> [w584]
            tunnel: w307 -> [w583]
            tunnel: w267 -> [w582]
            shift-right: [w581] -> _
            shift-left: errorcluster {"status"=FALSE, "code"=0, "source"=""} ("error out") -> [w580]
            stop <- w579 stop-if-true
            n209 = Get Queue Status(queue=w591, error in (no error)=w590) -> (queue out=w587:refnum<queue>, error out=w586:errorcluster, # elements in queue=w589:i32)  [unwired: 1 in, 5 out]
            n210 = Not Equal To 0?(x=w589) -> (x != 0?=w588:bool)
            n211 = case shown="True" w588 {
              tunnel: w587 -> [_ w610]
              tunnel: w586 -> [w592 w609]
              tunnel: [w592 w606] -> w585
              tunnel: w584 -> [_ w605]
              tunnel: w583 -> [_ w602]
              tunnel: w582 -> [_ w599]
              tunnel: [w593 w597] -> w581
              tunnel: w580 -> [w593 w596]
              frame False {
              }
              frame True {
                n212 = Dequeue Element(queue=w610, error in (no error)=w609) -> (element=w608:T7, error out=w606:errorcluster)  [unwired: 1 in, 2 out]
                n213 = call-poly <vilib>:"MT Matched Filter.vi"("input complex waveform"=w608, "matched filter coefficients"=w605, "samples per symbol (16)"=w602, "reset? (T)"=TRUE) -> ("output complex waveform"=w604:T7)  [unwired: 10 in, 1 out]
                n214 = call-poly <vilib>:"MT Align To Ideal Symbols.vi"("input complex waveform"=w604, "matched filter coefficients"=w605, "samples per symbol (16)"=w602, "reset? (T)"=TRUE) -> ("output complex waveform"=w603:T7, "error out"=w601:errorcluster)  [unwired: 9 in, 1 out]
                n215 = call <vilib>:"MT Decimate Oversampled Waveform.vi"("input complex waveform"=w603, "decimation factor"=w602, "error in (no error)"=w601, "reset? (T)"=TRUE) -> ("output complex waveform"=w600:T7)  [unwired: 10 in, 1 out]
                n216 = Unbundle(w600) -> ("Y"=w598:cdb[])  [unwired: 2 out]
                n217 = Enqueue Element(queue=w599, element=w598, error in (no error)=w596) -> (error out=w597:errorcluster)  [unwired: 1 in, 2 out]
              }
            }
            n218 = global read "var_stop.vi" "system stop"() -> (w579:bool)
          }
          n219 = while {
            tunnel: w266 -> [w623]
            shift-right: [w617] -> _
            shift-left: errorcluster {"status"=FALSE, "code"=0, "source"=""} ("error out") -> [w621]
            shift-right: [w615] -> _
            shift-left: cdb[] [] -> [w611]
            tunnel: w269 -> [w614]
            shift-right: [w613] -> _
            shift-left: errorcluster {"status"=FALSE, "code"=0, "source"=""} ("error out") -> [w612]
            stop <- w616 stop-if-true
            n220 = Get Queue Status(queue=w623, error in (no error)=w621) -> (queue out=w619:refnum<queue>, error out=w618:errorcluster, # elements in queue=w622:i32)  [unwired: 1 in, 5 out]
            n221 = Not Equal To 0?(x=w622) -> (x != 0?=w620:bool)
            n222 = case shown="True" w620 {
              tunnel: w619 -> [_ w646]
              tunnel: w618 -> [w625 w645]
              tunnel: [w625 w639] -> w617
              tunnel: w611 -> [w626 w643]
              tunnel: [w626 w633] -> w615
              tunnel: w614 -> [_ w629]
              tunnel: [w624 w628] -> w613
              tunnel: w612 -> [w624 w627]
              frame False {
              }
              frame True {
                n223 = Dequeue Element(queue=w646, error in (no error)=w645) -> (element=w644:T7, error out=w639:errorcluster)  [unwired: 1 in, 2 out]
                n224 = Unbundle(w644) -> ("t0"=w641:dbl, "dt"=w631:dbl, "Y"=w642:cdb[])
                n225 = Build Array (concatenate)(w643, w642) -> (w632:cdb[])
                n226 = Bundle(cluster=T7 {"t0"=0.0, "dt"=1.0, "Y"=[]} ("element"), "t0"=w641, "dt"=w631, "Y"=w632) -> (w640:T7)
                n227 = call "rx_ed.vi"("Wavefrom"=w640) -> ("first pulse"=w635:i32, "length"=w637:i32[], "start index"=w638:i32[])  [unwired: 8 in]
                n228 = for {
                  tunnel: w638 -> [w658] mode=indexing
                  tunnel: w637 -> [w653] mode=indexing
                  tunnel: [w660] -> w636
                  tunnel: w632 -> [w659]
                  tunnel: w631 -> [w656]
                  tunnel: w629 -> [w650]
                  shift-right: [w648] -> w628
                  shift-left: w627 -> [w649]
                  n229 = Array Subset(array=w659, index=w658, length=w653) -> (w657:cdb[])
                  n230 = Bundle(cluster=T7 {"t0"=0.0, "dt"=1.0, "Y"=[]} ("element"), "t0"=0.0, "dt"=w656, "Y"=w657) -> (w647:T7)
                  n231 = Add(x=w658, y=w653) -> (x+y=w660:i32)
                  n232 = Greater Or Equal?(x=w653, y=256) -> (x >= y?=w651:bool)
                  n233 = case shown="True" w651 {
                    tunnel: w650 -> [_ w665]
                    tunnel: w649 -> [w661 w664]
                    tunnel: [w661 w663] -> w648
                    tunnel: w647 -> [_ w662]
                    frame False {
                    }
                    frame True {
                      n234 = Enqueue Element(queue=w665, element=w662, error in (no error)=w664) -> (error out=w663:errorcluster)  [unwired: 1 in, 2 out]
                    }
                  }
                }
                n235 = Max & Min(x=w636, y=w635) -> (max(x,y)=w634:i32)  [unwired: 1 out]
                n236 = Array Subset(array=w632, index=w634) -> (w633:cdb[])  [unwired: 1 in]
              }
            }
            n237 = global read "var_stop.vi" "system stop"() -> (w616:bool)
          }
          n238 = while {
            shift-right: [w676] -> w316
            shift-left: w319 -> [w679]
            tunnel: w318 -> [w680]
            tunnel: [w677] -> w317
            tunnel: w266 -> [w675]
            shift-right: [w667] -> _
            shift-left: errorcluster {"status"=FALSE, "code"=0, "source"=""} ("error out") -> [w672]
            stop <- w666 stop-if-true
            n239 = call-poly <instrlib>:"niUSRP Fetch Rx Data (poly).vi"("session handle"=w680, "number of samples"="RX number of samples", "error in (no error)"=w679) -> ("session handle out"=w677:refnum<k15>, "data"=w668:cluster{"t0":dbl, "dt":dbl, "Y":cdb[]}, "error out"=w676:errorcluster)  [unwired: 9 in, 1 out]
            n240 = Get Queue Status(queue=w675, error in (no error)=w672) -> (queue out=w670:refnum<queue>, error out=w669:errorcluster, # elements in queue=w674:i32)  [unwired: 1 in, 5 out]
            n241 = Less?(x=w674, y=1000) -> (x < y?=w671:bool)
            n242 = case shown="True" w671 {
              tunnel: w670 -> [_ w685]
              tunnel: w669 -> [w681 w684]
              tunnel: w668 -> [_ w683]
              tunnel: [w681 w682] -> w667
              frame False {
              }
              frame True {
                n243 = Enqueue Element(queue=w685, element=w683, error in (no error)=w684) -> (error out=w682:errorcluster)  [unwired: 1 in, 2 out]
              }
            }
            n244 = global read "var_stop.vi" "system stop"() -> (w666:bool)
          }
          n245 = call <instrlib>:"niUSRP Abort.vi"("session handle"=w317, "error in (no error)"=w316) -> ("session handle out"=w321:refnum<k15>, "error out"=w320:errorcluster)  [unwired: 12 in]
          n246 = call <instrlib>:"niUSRP Close Session.vi"("session handle"=w321, "error in (no error)"=w320) -> ()  [unwired: 13 in, 1 out]
          n247 = while {
            tunnel: w270 -> [w350]
            shift-right: [w344] -> _
            shift-left: errorcluster {"status"=FALSE, "code"=0, "source"=""} ("error out") -> [w348]
            shift-right: [w341] -> _
            shift-left: 0 -> [w342]
            shift-right: [w343] -> w282
            shift-left: cluster{"counter":u32, u8[]}[] [] -> [w337]
            stop <- w339 stop-if-true
            n248 = Get Queue Status(queue=w350, error in (no error)=w348) -> (queue out=w346:refnum<queue>, error out=w345:errorcluster, # elements in queue=w349:i32)  [unwired: 1 in, 5 out]
            n249 = Not Equal To 0?(x=w349) -> (x != 0?=w347:bool)
            n250 = case shown="True" w347 {
              tunnel: w346 -> [_ w378]
              tunnel: w345 -> [w354 w377]
              tunnel: [w354 w366] -> w344
              tunnel: [w351 w364] -> w343
              tunnel: w342 -> [w353 w367]
              tunnel: [w353 w362] -> w341
              tunnel: [FALSE w363] -> w338
              tunnel: w337 -> [w351 w355]
              frame False {
              }
              frame True {
                n251 = Array Size(array=w355) -> (size(s)=w370:i32)
                n252 = Dequeue Element(queue=w378, error in (no error)=w377) -> (element=w365:cluster{"counter":u32, "bitstream":bool[]}, error out=w366:errorcluster)  [unwired: 1 in, 2 out]
                n253 = Unbundle(w365) -> ("counter"=w371:u32, "bitstream"=w357:bool[])
                n254 = global read "glb_ackTable.vi" "ACK table"() -> (w372:bool[])
                n255 = Array Size(array=w372) -> (size(s)=w368:i32)
                n256 = Index Array(array=w372, index=w371) -> (element=w376:bool)
                n257 = Not Equal?(x=w368, y=w370) -> (x != y?=w369:bool)
                n258 = Not(x=w376) -> (.not. x?=w375:bool)
                n259 = Less?(x=w371, y=w368) -> (x < y?=w374:bool)
                n260 = And(x=w375, y=w374) -> (x .and. y?=w373:bool)
                n261 = case shown="False" w369 {
                  tunnel: w368 -> [w380 w383]
                  tunnel: [w380 w383] -> w361
                  tunnel: w355 -> [w379 _]
                  tunnel: [w379 w381] -> w356
                  frame False {
                  }
                  frame True {
                    n262 = Initialize Array(cluster{"counter":u32, u8[]} {"counter"=0, []} ("cluster"), w383) -> (w381:cluster{"counter":u32, u8[]}[])
                  }
                }
                n263 = case shown="False" w373 {
                  tunnel: w372 -> [_ w401]
                  tunnel: w371 -> [_ w386]
                  tunnel: w367 -> [w385 w398]
                  tunnel: [w385 w397] -> w362
                  tunnel: [w384 w387] -> w364
                  tunnel: w357 -> [_ w396]
                  tunnel: w356 -> [w384 w388]
                  frame False {
                  }
                  frame True {
                    w393 = 8 ("y")
                    n264 = Array Size(array=w396) -> (size(s)=w395:i32)
                    n265 = Replace Array Subset(array=w401, new element=TRUE, index=w386) -> (w399:bool[])
                    n266 = Quotient & Remainder(x=w395, y=w393) -> (floor(x/y)=w394:i32)  [unwired: 1 out]
                    n267 = Increment(x=w398) -> (x+1=w397:i32)
                    n268 = Reshape Array(w396, w394, w393) -> (w392:bool[][])
                    n269 = global write "glb_ackTable.vi" "ACK table"(w399) -> ()
                    n270 = for {
                      tunnel: w392 -> [w404] mode=indexing
                      tunnel: [w402] -> w391 mode=indexing
                      n271 = Boolean Array To Number(Boolean array=w404) -> (number=w403:u32)
                      n272 = To Unsigned Byte Integer(number=w403) -> (unsigned 8bit integer=w402:u8)
                    }
                    n273 = Bundle(cluster=cluster{"counter":u32, u8[]} {"counter"=0, []}, "counter"=w386, w391) -> (w390:cluster{"counter":u32, u8[]})
                    n274 = Replace Array Subset(array=w388, new element=w390, index=w386) -> (w387:cluster{"counter":u32, u8[]}[])
                  }
                }
                n275 = Equal?(x=w362, y=w361) -> (x = y?=w363:bool)
                n276 = Divide(x=w362, y=w361) -> (x/y=w360:dbl)
                n277 = Multiply(x=100.0, y=w360) -> (x*y=→"Download progress":dbl)
              }
            }
            n278 = global read "var_stop.vi" "system stop"() -> (w340:bool)
            n279 = global write "glb_complete.vi" "Complete"(w338) -> ()
            n280 = Compound Arithmetic op=OR(w338, w340) -> (w339:bool)
          }
        }
        frame Error {
        }
      }
    }
    frame #2 {
      n281 = Release Queue(queue=w827) -> ()  [unwired: 2 in, 3 out]
      n282 = Release Queue(queue=w828) -> ()  [unwired: 2 in, 3 out]
      n283 = Release Queue(queue=w826) -> ()  [unwired: 2 in, 3 out]
      n284 = for {
        tunnel: [w878] -> w842 mode=indexing
        tunnel: [w877] -> w839 mode=concatenating
        tunnel: w841 -> [w876] mode=indexing
        n285 = Unbundle(w876) -> (w877:u8[])  [unwired: 1 out]
        n286 = Array Size(array=w877) -> (size(s)=w878:i32)
      }
      n287 = Unbundle(w840) -> ("use 24bit?"=w838:bool, "dimension"=w837:i32[], "top left"=w834:cluster{"x":i16, "y":i16}, "colors"=w836:u32[], "mask"=w835:u8[])
      n288 = Release Queue(queue=w829) -> ()  [unwired: 2 in, 3 out]
      n289 = Release Queue(queue=w830) -> ()  [unwired: 2 in, 3 out]
      n290 = Release Queue(queue=w831) -> ()  [unwired: 2 in, 3 out]
      n291 = Add Array Elements(numeric array=w842) -> (sum=→"total bytes RX":i32)
      n292 = case shown="True" w838 {
        tunnel: w839 -> [w844 w861]
        tunnel: w837 -> [w854 w870]
        tunnel: w836 -> [w848 w864]
        tunnel: w835 -> [w847 w865]
        tunnel: w834 -> [w846 w863]
        tunnel: [w845 w862] -> w833
        frame False {
          n293 = Index Array(array=w854, index=1) -> (element=w850:i32)
          n294 = Index Array(array=w854, index=0) -> (element=w851:i32)
          n295 = Reshape Array(w844, w851, w850) -> (w849:u8[][])
          n296 = call <vilib>:"Flatten Pixmap.vi"("mask"=w847, "colors"=w848, "top left"=w846, "8-bit pixmap"=w849) -> ("image data"=w845:T8)  [unwired: 7 in]
        }
        frame True {
          w857 = 24 ("y")
          # "24 bits color image"
          n297 = for {
            tunnel: w861 -> [w875] mode=indexing
            tunnel: [w874] -> w859 mode=concatenating
            n298 = Number To Boolean Array(number=w875) -> (Boolean array=w874:bool[])
          }
          n299 = Array Size(array=w859) -> (size(s)=w860:i32)
          n300 = Index Array(array=w870, index=0) -> (element=w868:i32)
          n301 = Index Array(array=w870, index=1) -> (element=w867:i32)
          n302 = Quotient & Remainder(x=w860, y=w857) -> (floor(x/y)=w858:i32)  [unwired: 1 out]
          n303 = Reshape Array(w859, w858, w857) -> (w856:bool[][])
          n304 = for {
            tunnel: w856 -> [w873] mode=indexing
            tunnel: [w872] -> w855 mode=indexing
            n305 = Boolean Array To Number(Boolean array=w873) -> (number=w872:u32)
          }
          n306 = Reshape Array(w855, w868, w867) -> (w866:u32[][])
          n307 = call <vilib>:"Flatten Pixmap.vi"("mask"=w865, "colors"=w864, "top left"=w863, "24-bit pixmap"=w866) -> ("image data"=w862:T8)  [unwired: 7 in]
        }
      }
      n308 = call <vilib>:"Draw Flattened Pixmap.vi"("image data"=w833) -> ("new picture"=→"Received Image":picture)  [unwired: 8 in]
    }
  }
  n309 = Initialize Array(cdb 0.0+0.0i, 20000 ("dimension size")) -> (w11:cdb[])
